vi "toggle.vi"() -> ()   [LabVIEW 2017]
panel:
  out "toggle":bool
  in  "control":bool
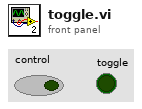
[diagram p1: front panel]
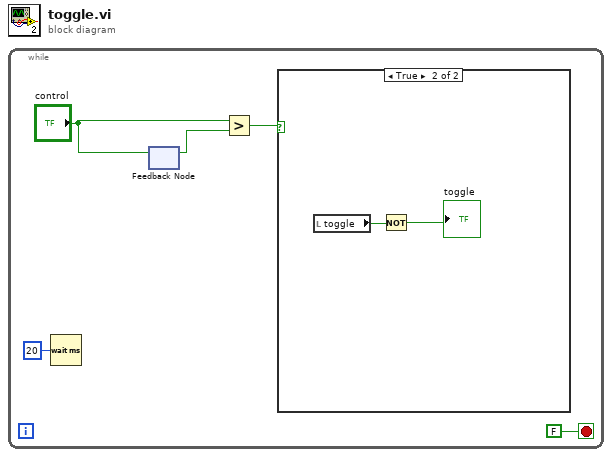
[diagram p0: block diagram]
diagram:
  n1 = while {
    stop <- FALSE stop-if-true
    n2 = Wait (ms)(milliseconds to wait=u32 20) -> ()  [unwired: 1 out]
    n3 = feedback #1() -> (w5:bool)  [unwired: 1 in]
    n4 = feedback-in #1("control") -> ()
    n5 = Greater?(x="control", y=w5) -> (0:w3:bool)
    n6 = case shown="True" w3 {
      frame False {
      }
      frame True {
        n7 = local read "toggle"() -> (w7:bool)
        n8 = Not(x=w7) -> (.not. x?=→"toggle":bool)
      }
    }
  }
